vi "LCDset.vi"(10 "in in LINE2":string, 11 "in LINE1":string) -> (1 "Line1":string, 2 "unsigned byte array":u8[](array[numeric]), 3 "unsigned byte array 2":u8[](array[numeric]), 5 "Line2":string)   [LabVIEW 2019]
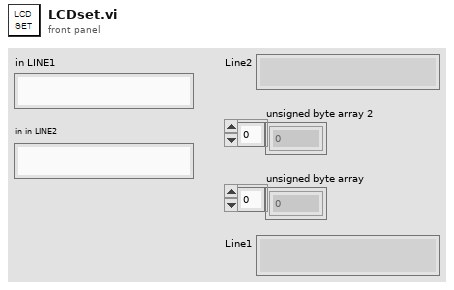
[diagram p1: front panel]
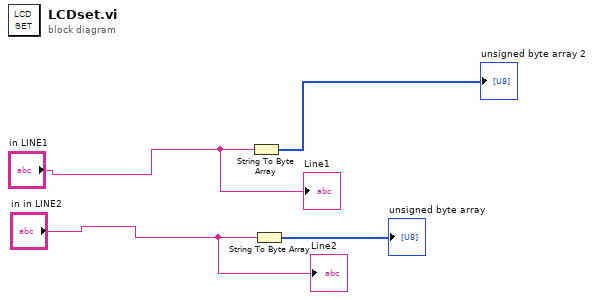
[diagram p0: block diagram]
diagram:
  n1 = String To Byte Array(string="in LINE1") -> (unsigned byte array=→"unsigned byte array 2":u8[])
  n2 = String To Byte Array(string="in in LINE2") -> (unsigned byte array=→"unsigned byte array":u8[])
  "Line1" <- "in LINE1"
  "Line2" <- "in in LINE2"
